vi "PCert-Container-UI.vi"(11 "error constant":errorcluster) -> (15 "error constant 2":errorcluster)   [LabVIEW 2013, in "PCert-Container-UI.lvclass"]
uses:
  PCert-Container-UI.lvclass
  PCert-Container-UI.lvclass/PCert-Container-UI.ctl
  ftw-dataflow/Actor/src/Connector/FTW-ActorConnector.lvclass
  ftw-dataflow/Actor/src/Message/Request/FTW-Message-IncomingRequest.lvclass
  ERP-Glue/PCert-Glue-TreeItem.ctl
  Actors/Globals/Global-SystemSettings.vi
  ftw-dataflow/Actor/src/Instance/FTW-ActorInstance.lvclass
  ftw-dataflow/Actor/src/Ether/FTW-Ether.lvclass
  ERP-ConfigPageNewFeather/PCert-ConfigPageNF.lvclass
  <resource>/Framework/Providers/Wirebird Labs LLC/Deploy/Support/Update Service/Deploy-UpdateService.lvclass
panel:
  in  "UI_Tree_Navigation":string(tree) caption="Navigation Tree"
  in  "Shutdown":bool
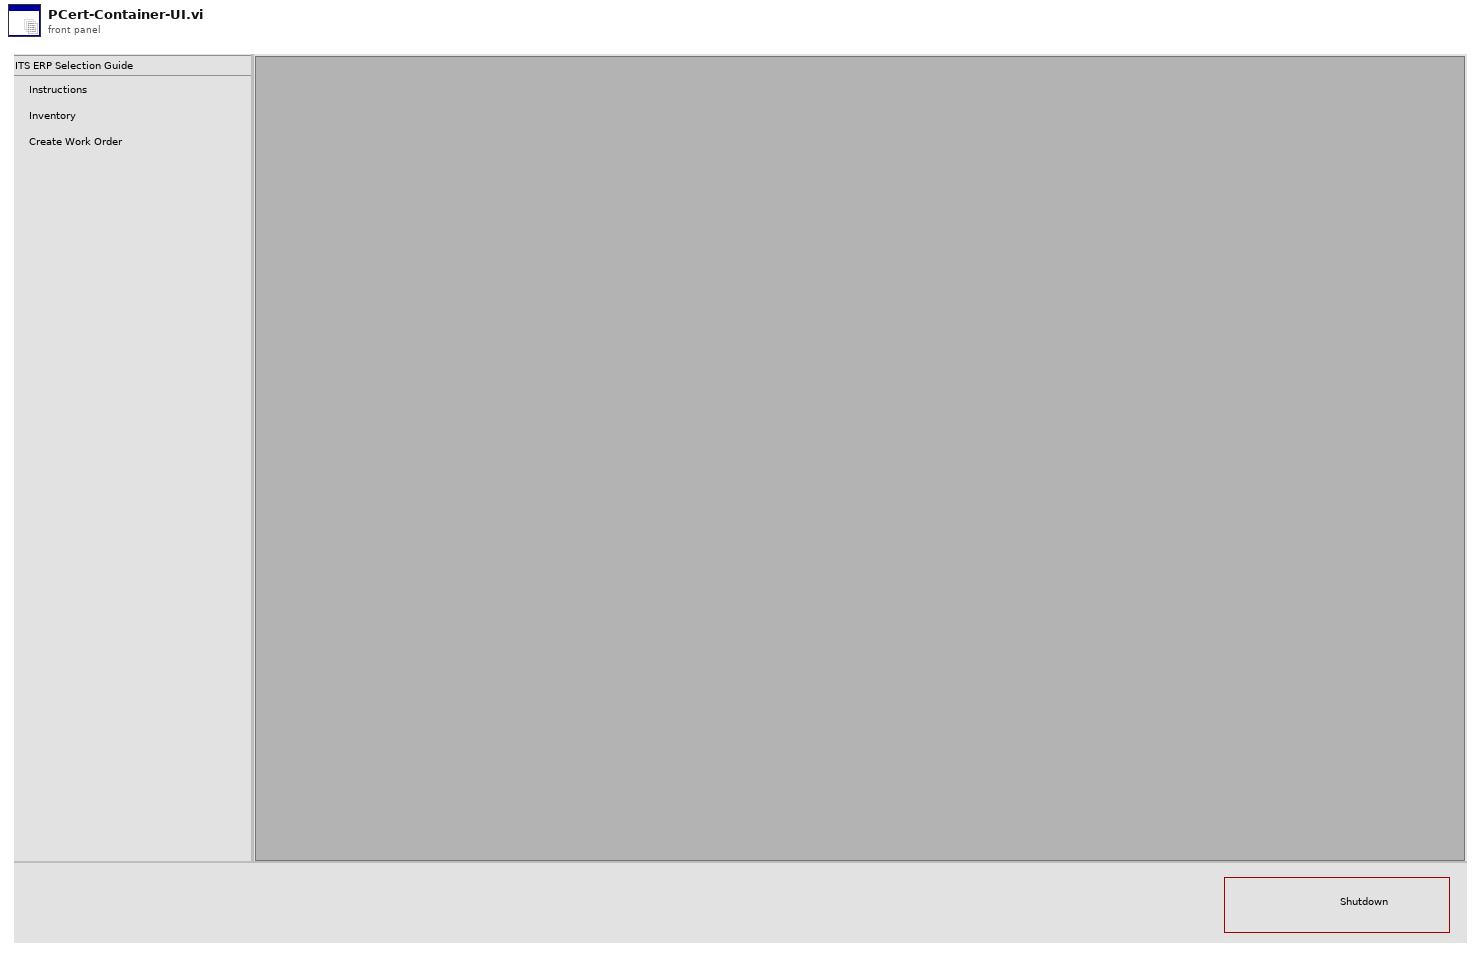
[diagram p1: front panel]
types:
  T1 = typedef "PCert-Glue-TreeItem.ctl" = cluster{"Tag":string, "Parent":string, "Add to Top of Parent":bool, "Type":string, "Indent":i32, "Child Only":bool, "First Cell":string, "Next Cells":string[]}
  T2 = cluster{"Incoming Requests":refnum<event-registration>, "Update Service Event Registration":refnum<event-registration>}
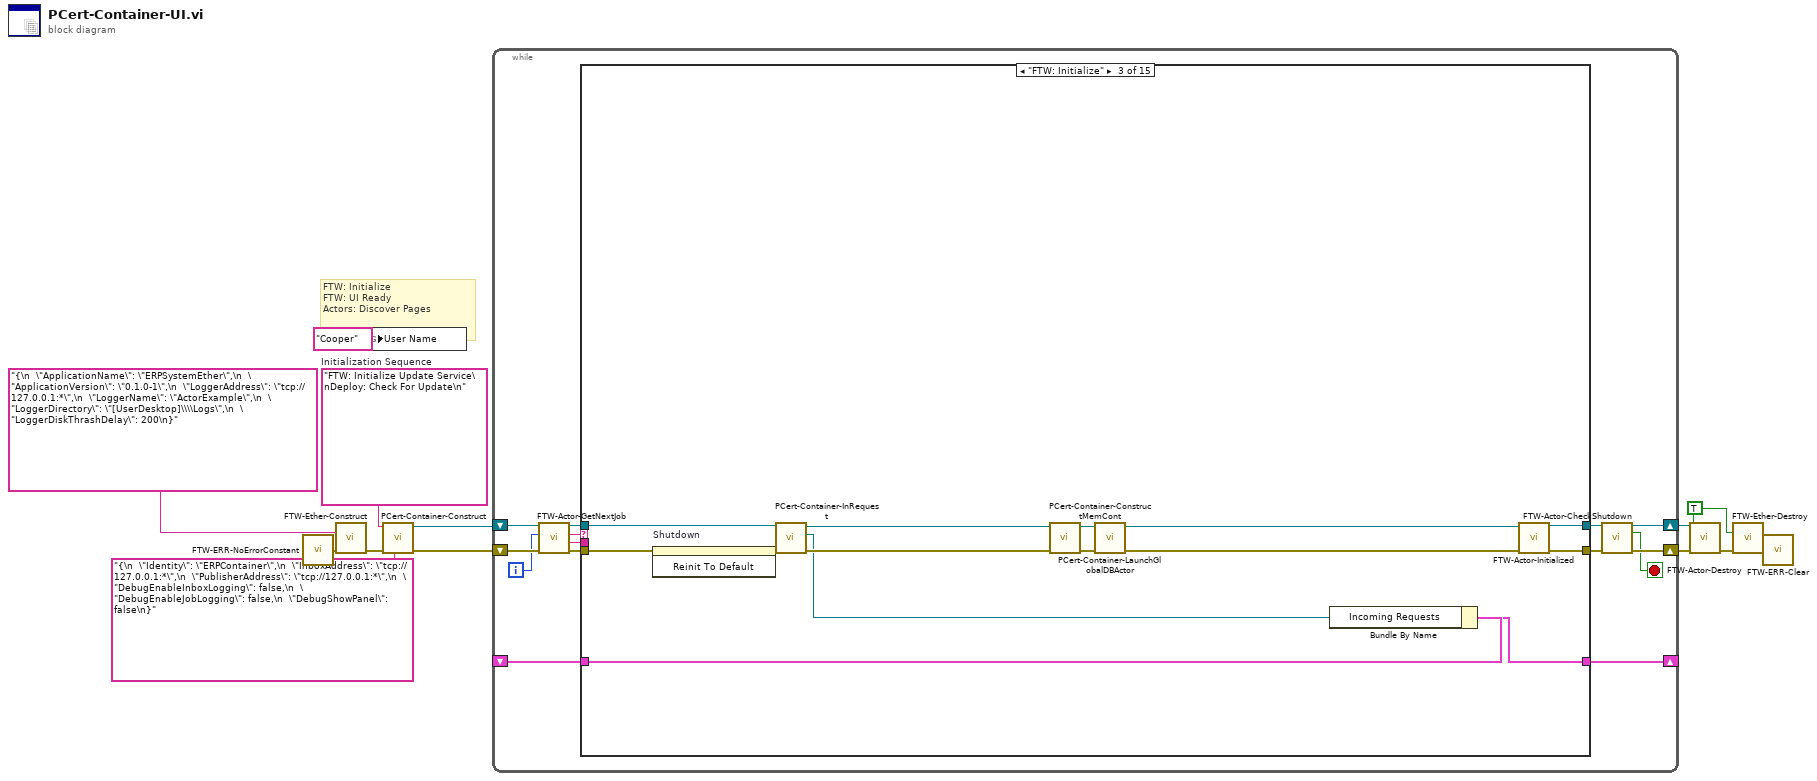
[diagram p0: block diagram]
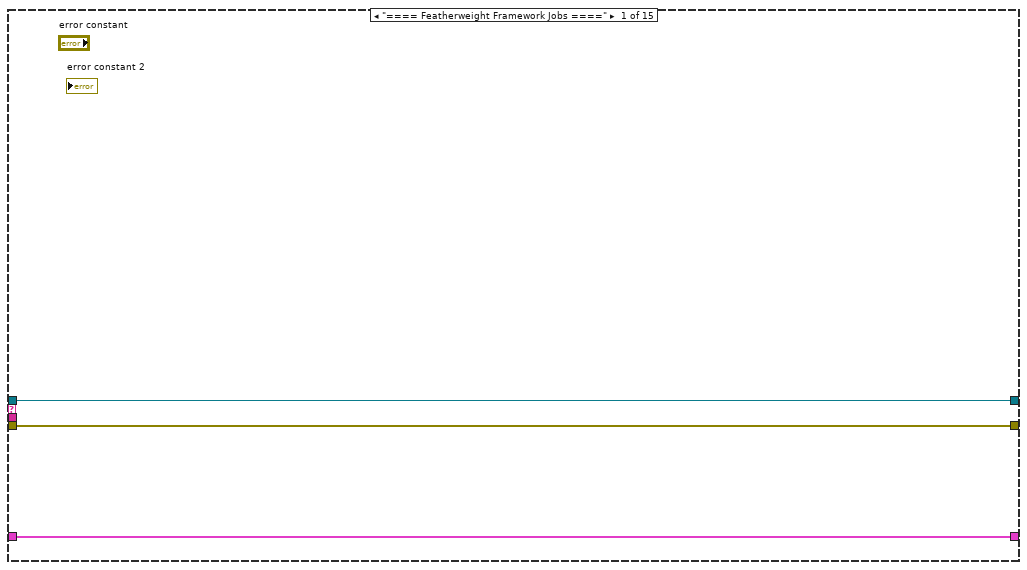
[diagram p2: hidden frame]
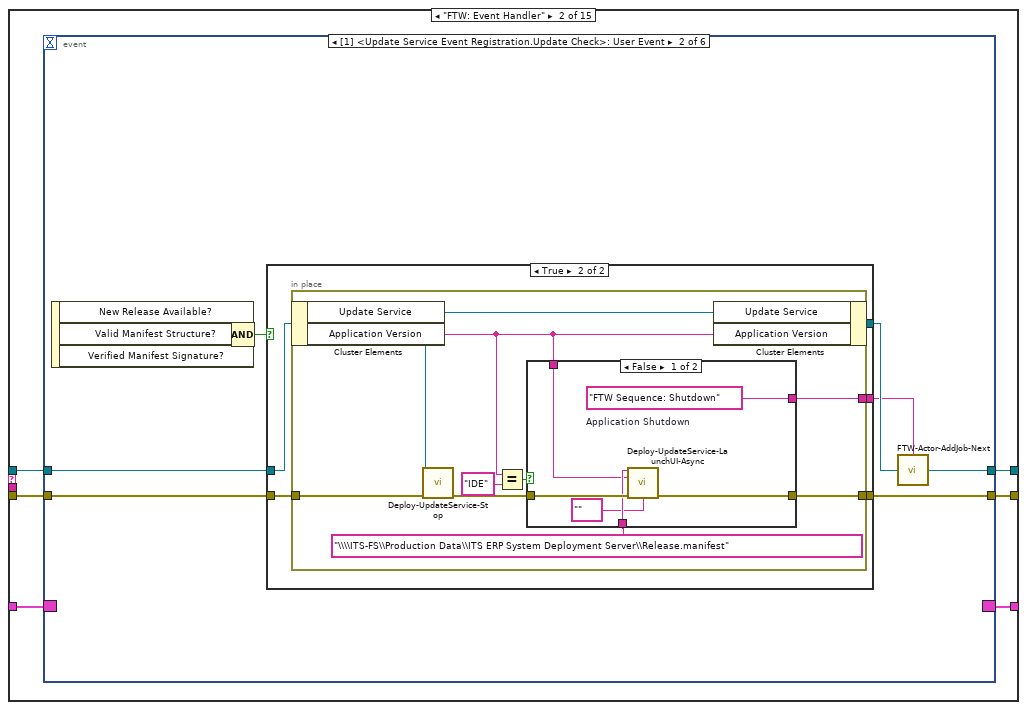
[diagram p3: hidden frame]
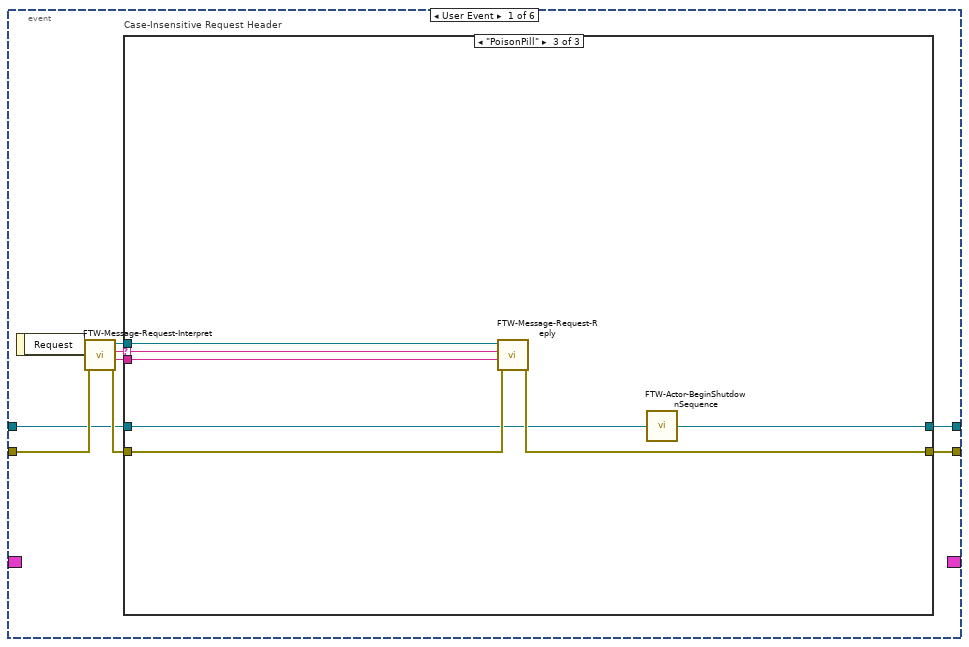
[diagram p4: hidden frame]
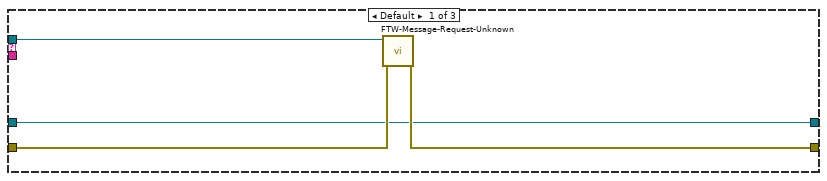
[diagram p5: hidden frame]
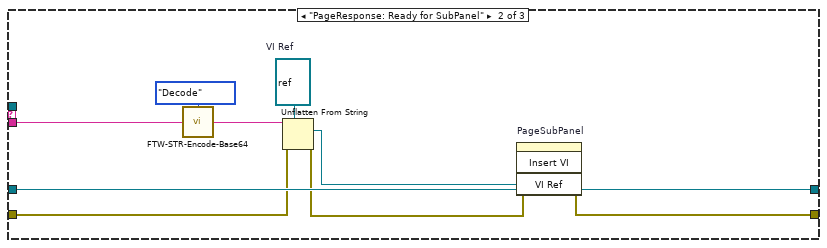
[diagram p6: hidden frame]
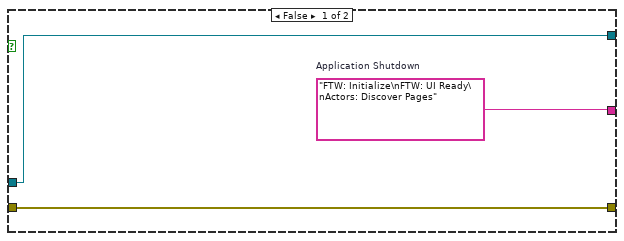
[diagram p7: hidden frame]
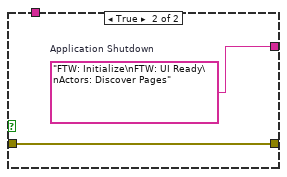
[diagram p8: hidden frame]
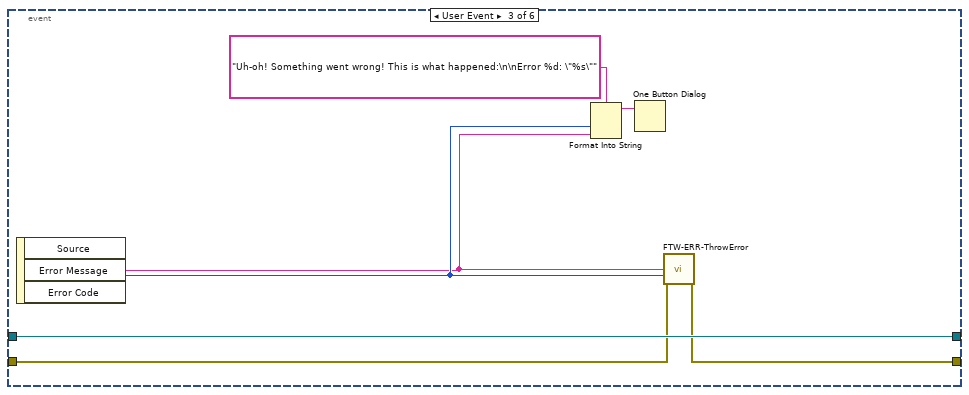
[diagram p9: hidden frame]
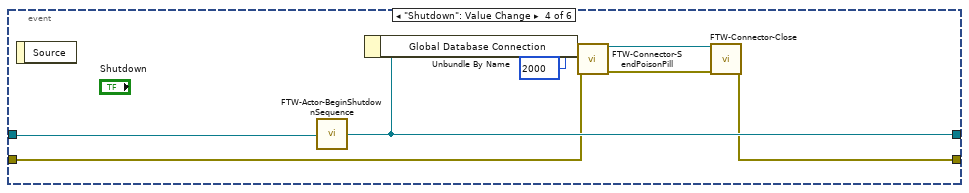
[diagram p10: hidden frame]
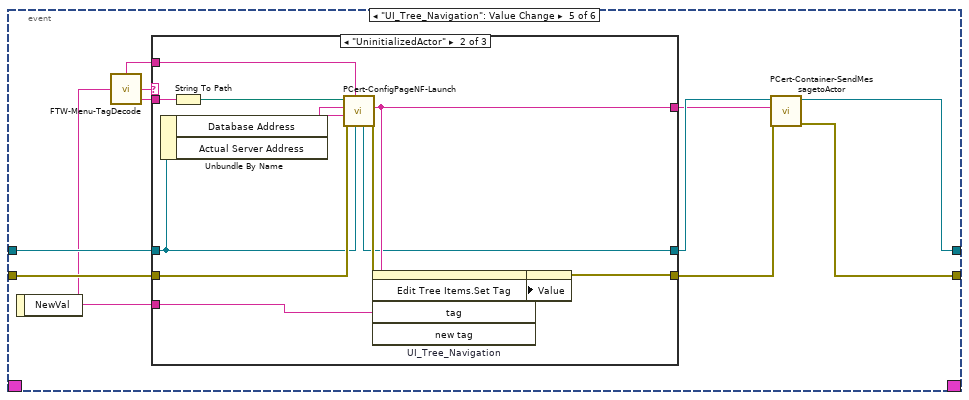
[diagram p11: hidden frame]
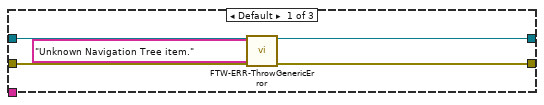
[diagram p12: hidden frame]
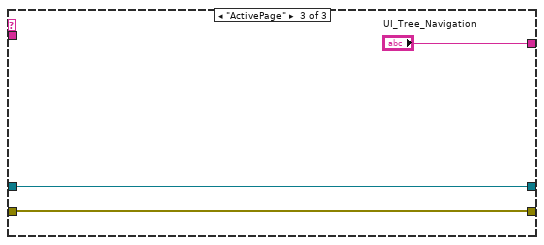
[diagram p13: hidden frame]
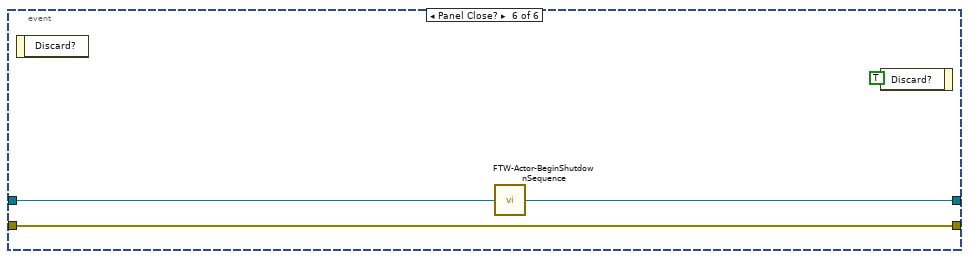
[diagram p14: hidden frame]
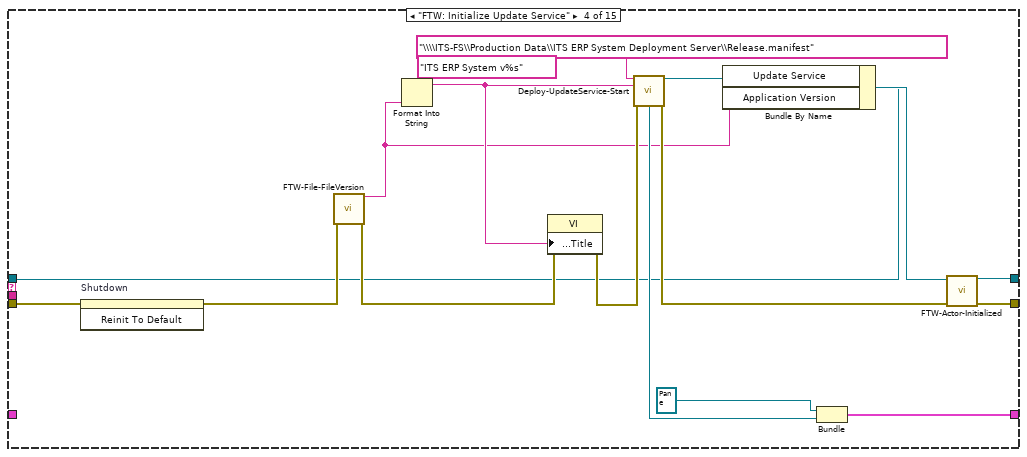
[diagram p15: hidden frame]
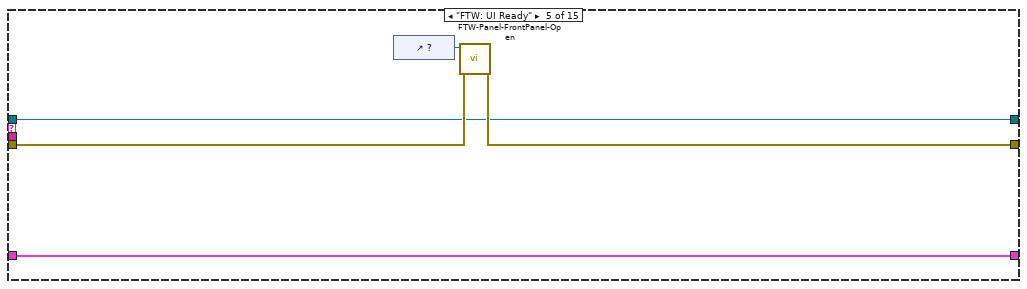
[diagram p16: hidden frame]
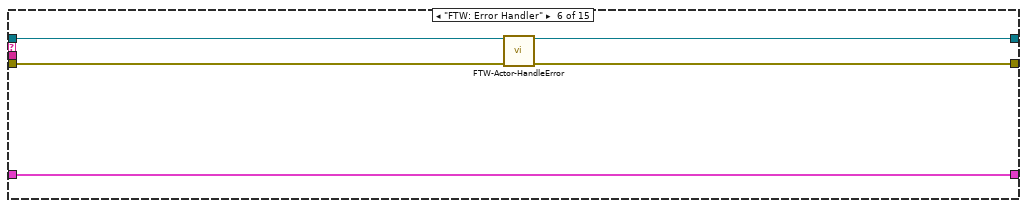
[diagram p17: hidden frame]
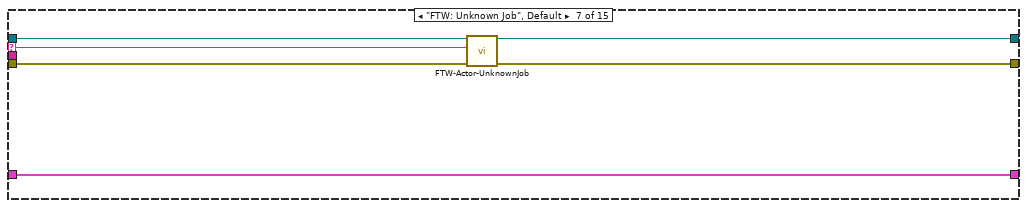
[diagram p18: hidden frame]
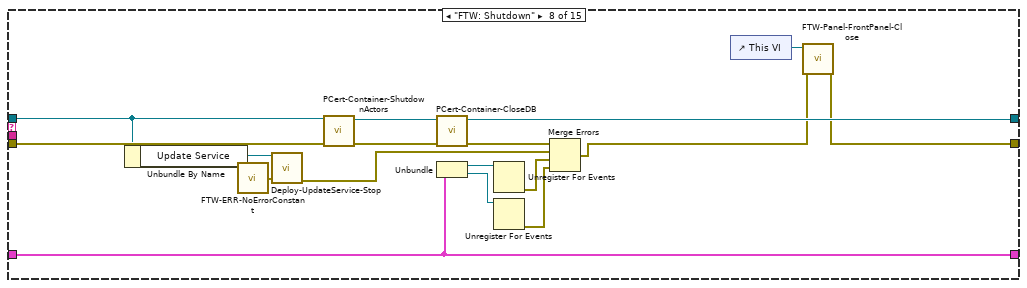
[diagram p19: hidden frame]
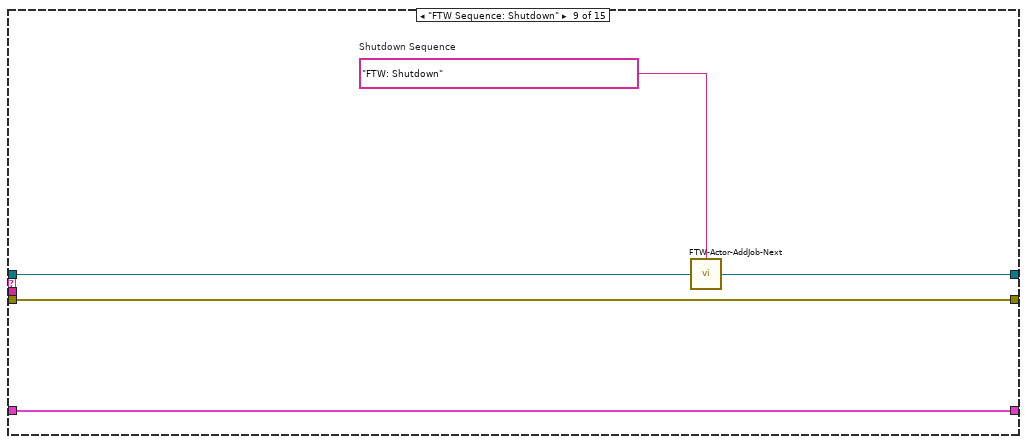
[diagram p20: hidden frame]
diagram:
  w2 = TRUE ("Force Destroy?")
  w6 = "FTW: Initialize Update Service\nDeploy: Check For Update\n"  # Initialization Sequence
  # "FTW: Initialize\nFTW: UI Ready\nActors: Discover Pages"
  n1 = call "FTW-ERR-NoErrorConstant.vi"() -> ("no error"=w4:errorcluster)
  n2 = call "FTW-Ether-Construct.vi"("FTW Ether Configuration"="{\n  \"ApplicationName\": \"ERPSystemEther\",\n  \"ApplicationVersion\": \"0.1.0-1\",\n  \"LoggerAddress\": \"tcp://127.0.0.1:*\",\n  \"LoggerName\": \"ActorExample\",\n  \"LoggerDirectory\": \"[UserDesktop]\\\\Logs\",\n  \"LoggerDiskThrashDelay\": 200\n}", "error in"=w4) -> ("error out"=w5:errorcluster)  [unwired: 13 in]
  n3 = global write "Global-SystemSettings.vi" "User Name"("Cooper" ("User Name")) -> ()
  n4 = call "PCert-Container-Construct.vi"("FTW Actor Instance Configuration"="{\n  \"Identity\": \"ERPContainer\",\n  \"InboxAddress\": \"tcp://127.0.0.1:*\",\n  \"PublisherAddress\": \"tcp://127.0.0.1:*\",\n  \"DebugEnableInboxLogging\": false,\n  \"DebugEnableJobLogging\": false,\n  \"DebugShowPanel\": false\n}", "error in (no error)"=w5, "Initialization Sequence"=w6) -> ("error out"=w8:errorcluster, "ERP-Container-UI out"=w9:refnum<class "PCert-Container-UI.lvclass">)  [unwired: 7 in]
  n5 = while {
    shift-right: [w18] -> w12
    shift-left: w8 -> [w25]
    shift-right: [w15] -> _
    shift-left: _ -> [w14]
    shift-right: [w20] -> w13
    shift-left: w9 -> [w27]
    i -> [w16]
    stop <- w17 stop-if-true
    n6 = call "FTW-Actor-GetNextJob.vi"("error in"=w25, "Jobs Performed"=w16, "FTW Actor Instance"=w27) -> ("error out"=w24:errorcluster, "Job Data"=w22:string, "Job Name"=w23:string, "FTW Actor Instance out"=w26:refnum<class "PCert-Container-UI.lvclass">)  [unwired: 5 in]
    n7 = case shown="\"FTW: Initialize\"" w23 {
      selector: w23 -> [_ _ _ _ _ _ w193 _ _ _ _ _ _ _ _]
      tunnel: [w29 w36 w164 w181 w185 w189 w196 w207 w216 w224 w228 w231 w234 w255 w259] -> w19
      tunnel: w24 -> [w29 w35 w158 w179 w187 w188 w197 w206 w216 w224 w228 w231 w245 w255 w260]
      tunnel: w14 -> [w30 w31 w154 _ w183 w192 w198 w215 w220 w225 w227 w230 w247 w254 w262]
      tunnel: [w30 w32 w152 w180 w183 w192 w198 w215 w220 w225 w227 w230 w247 w254 w262] -> w15
      tunnel: w22 -> [_ _ _ _ _ _ _ _ _ _ _ _ _ _ _]
      tunnel: [w28 w34 w165 w182 w184 w190 w194 w212 w218 w222 w226 w229 w246 w253 w257] -> w21
      tunnel: w26 -> [w28 w33 w161 w169 w184 w191 w195 w202 w219 w223 w226 w229 w246 w253 w261]
      frame "==== Featherweight Framework Jobs ====" {
      }
      frame "FTW: Event Handler" {
        n8 = event shown="[1] <Update Service Event Registration.Update Check>: User Event" {
          selector: w31 -> [_ _ _ _ _ _]
          dyn-events: [_ _ _ _ _ _] -> w32
          timeout: _ -> [_ _ _ _ _ _]
          tunnel: [w42 w69 w103 w113 w118 w150] -> w36
          tunnel: w35 -> [w43 w74 w104 w108 w123 w150]
          tunnel: [w41 w66 w107 w114 w117 w148] -> w34
          tunnel: w33 -> [w40 w75 w107 w115 w124 w149]
          event User Event {
            n9 = event-data() -> ("Request"=w44:refnum<class "FTW-Message-IncomingRequest.lvclass">)  [unwired: 1 in]
            n10 = call "FTW-Message-Request-Interpret.vi"("error in"=w43, "FTW Incoming Request"=w44) -> ("error out"=w45:errorcluster, "Request Body"=w38:string, "Request Header"=w39:string, "FTW Incoming Request out"=w37:refnum<class "FTW-Message-IncomingRequest.lvclass">)  [unwired: 6 in]
            n11 = case "Case-Insensitive Request Header" shown="\"PoisonPill\"" w39 {
              selector: w39 -> [_ _ w61]
              tunnel: [w48 w54 w63] -> w42
              tunnel: w45 -> [w49 w53 w64]
              tunnel: [w46 w58 w65] -> w41
              tunnel: w40 -> [w46 w58 w62]
              tunnel: w38 -> [_ w52 w60]
              tunnel: w37 -> [w47 _ w59]
              frame Default {
                n12 = call "FTW-Message-Request-Unknown.vi"("error in"=w49, "FTW Incoming Request"=w47) -> ("error out"=w48:errorcluster)  [unwired: 9 in]
              }
              frame "PageResponse: Ready for SubPanel" {
                w57 = refnum<vi> refnum  # VI Ref
                n13 = call "FTW-STR-Encode-Base64.vi"("Input"=w52, "Direction"=enum16{"Encode", "Decode"}."Decode") -> ("Output"=w50:string)
                n14 = Unflatten From String(type=w57, binary string=w50, error in (no error)=w53) -> (value=w56:refnum<vi>, error out=w55:errorcluster)  [unwired: 2 in, 1 out]
                n15 = invoke on="PageSubPanel" class="SubPnl" method="Insert VI"(error in=w55, "VI Ref"=w56) -> (error out=w54:errorcluster)  [unwired: 2 in, 3 out]
              }
              frame "PoisonPill" {
                n16 = call "FTW-Message-Request-Reply.vi"("error in"=w64, "Response Body"=w60, "Response Header"=w61, "FTW Incoming Request"=w59) -> ("error out"=w63:errorcluster)  [unwired: 6 in, 1 out]
                n17 = call "FTW-Actor-BeginShutdownSequence.vi"("FTW Actor Instance"=w62) -> ("FTW Actor Instance out"=w65:refnum<class "PCert-Container-UI.lvclass">)  [unwired: 3 in]
              }
            }
          }
          event User Event {
            n18 = event-data() -> ("New Release Available?"=w73:bool, "Valid Manifest Structure?"=w72:bool, "Verified Manifest Signature?"=w71:bool)  [unwired: 1 in]
            n19 = Compound Arithmetic op=AND(w73, w72, w71) -> (w70:bool)
            n20 = case shown="True" w70 {
              tunnel: w75 -> [w78 w83]
              tunnel: w74 -> [w77 w82]
              tunnel: [w78 w81] -> w68
              tunnel: [w77 w80] -> w69
              tunnel: [w76 w79] -> w67
              frame False {
                w76 = "FTW: Initialize\nFTW: UI Ready\nActors: Discover Pages"  # Application Shutdown
              }
              frame True {
                n21 = in-place {
                  in-place-border: w82 -> [w92]
                  in-place-border: [w88] -> w80
                  in-place-border: [w84] -> w79
                  n22 = in-place-cluster #1(w83) -> ("Update Service"=w91:refnum<class "Deploy-UpdateService.lvclass">, "Application Version"=w86:string)
                  n23 = call <resource>:"Deploy-UpdateService-Stop.vi"("Update Service"=w91, "error in"=w92) -> ("error out"=w90:errorcluster)  [unwired: 13 in]
                  n24 = Equal?(x=w86, y="IDE") -> (x = y?=w87:bool)
                  n25 = case shown="False" w87 {
                    tunnel: w90 -> [w98 w100]
                    tunnel: "\\\\ITS-FS\\Production Data\\ITS ERP System Deployment Server\\Release.manifest" ("Manifest URI") -> [w97 _]
                    tunnel: [w95 w100] -> w88
                    tunnel: w86 -> [w94 _]
                    tunnel: [w93 w99] -> w84
                    frame False {
                      w93 = "FTW Sequence: Shutdown"  # Application Shutdown
                      n26 = call <resource>:"Deploy-UpdateService-LaunchUI-Async.vi"("Manifest URI"=w97, "Current Release Version"=w94, "error in"=w98, "Installer Command Line Parameters"="") -> ("error out"=w95:errorcluster)  [unwired: 10 in, 1 out]
                    }
                    frame True {
                      w99 = "FTW: Initialize\nFTW: UI Ready\nActors: Discover Pages"  # Application Shutdown
                    }
                  }
                  n27 = in-place-cluster #1("Update Service"=w91, "Application Version"=w86) -> (w81:refnum<class "PCert-Container-UI.lvclass">)
                }
              }
            }
            n28 = call "FTW-Actor-AddJob-Next.vi"("Add Next in Job Queue"=w67, "FTW Actor Instance"=w68) -> ("FTW Actor Instance out"=w66:refnum<class "PCert-Container-UI.lvclass">)  [unwired: 2 in]
          }
          event User Event {
            n29 = event-data() -> ("Error Message"=w101:string, "Error Code"=w102:i32)  [unwired: 1 in, 1 out]
            n30 = Format Into String(format string="Uh-oh! Something went wrong! This is what happened:\n\nError %d: \"%s\"", w102, w101) -> (resulting string=w106:string)  [unwired: 2 in, 1 out]
            n31 = One Button Dialog(message=w106) -> ()  [unwired: 1 in, 1 out]
            n32 = call "FTW-ERR-ThrowError.vi"("Error Message"=w101, "Error Code"=w102, "error in"=w104) -> ("error out"=w103:errorcluster)  [unwired: 12 in]
          }
          event "Shutdown": Value Change {
            n33 = event-data() -> ()  [unwired: 1 in, 1 out]
            n34 = call "FTW-Actor-BeginShutdownSequence.vi"("FTW Actor Instance"=w115) -> ("FTW Actor Instance out"=w114:refnum<class "PCert-Container-UI.lvclass">)  [unwired: 3 in]
            n35 = Unbundle By Name(w114) -> ("Global Database Connection"=w112:refnum<class "FTW-ActorConnector.lvclass">)
            n36 = call-dynamic "FTW-Connector-SendPoisonPill.vi"("FTW Actor Connector"=w112, "Timeout"=2000, "error in"=w108) -> ("FTW Actor Connector out"=w111:refnum<class "FTW-ActorConnector.lvclass">, "error out"=w110:errorcluster)  [unwired: 8 in, 3 out]
            n37 = call-dynamic "FTW-Connector-Close.vi"("FTW Actor Connector"=w111, "error in"=w110) -> ("error out"=w113:errorcluster)  [unwired: 13 in]
          }
          event "UI_Tree_Navigation": Value Change {
            n38 = event-data() -> ("NewVal"=w122:string)  [unwired: 1 in]
            n39 = call "FTW-Menu-TagDecode.vi"("Menu Item Tag"=w122) -> ("Actor Name"=w116:string, "Command"=w126:string, "Payload"=w125:string)  [unwired: 1 out]
            n40 = case shown="\"UninitializedActor\"" w126 {
              tunnel: w125 -> [_ w142 _]
              tunnel: w124 -> [w130 w135 w146]
              tunnel: [w130 w131 w146] -> w121
              tunnel: w123 -> [w129 w144 w145]
              tunnel: [w128 w132 w145] -> w119
              tunnel: w122 -> [_ w139 _]
              tunnel: [_ w133 "UI_Tree_Navigation"] -> w120
              tunnel: w116 -> [_ w136 _]
              frame Default {
                n41 = call "FTW-ERR-ThrowGenericError.vi"("Error Message"="Unknown Navigation Tree item.", "error in"=w129) -> ("error out"=w128:errorcluster)  [unwired: 13 in]
              }
              frame "UninitializedActor" {
                n42 = Unbundle By Name(w135) -> ("Database Address"=w134:string, "Actual Server Address"=w143:string)
                n43 = String To Path(string=w142) -> (path=w141:path)
                n44 = call "PCert-ConfigPageNF-Launch.vi"("ERP-Container-UI in"=w135, "Actor Name"=w136, "error in (no error)"=w144, "Container Address"=w143, "Database Address"=w134, "Configuration Page VI Filepath"=w141) -> ("error out"=w140:errorcluster, "PageID"=w133:string, "ERP-Container-UI out"=w131:refnum<class "PCert-Container-UI.lvclass">)  [unwired: 3 in]
                n45 = invoke on="UI_Tree_Navigation" class="Tree (strict)" method="Edit Tree Items.Set Tag"(error in=w140, "tag"=w139, "new tag"=w133) -> (error out=w138:errorcluster, "Edit Tree Items:Set Tag"=w137:string)  [unwired: 2 in, 3 out]
                n46 = property on="UI_Tree_Navigation" class="Tree (strict)"(error in=w138, "Value"=w137) -> (error out=w132:errorcluster)  [unwired: 1 in, 1 out]
              }
              frame "ActivePage" {
              }
            }
            n47 = call "PCert-Container-SendMessagetoActor.vi"("error in (no error)"=w119, "ActorID"=w120, "ERP-Container-UI in"=w121) -> ("error out"=w118:errorcluster, "ERP-Container-UI out"=w117:refnum<class "PCert-Container-UI.lvclass">)  [unwired: 7 in]
          }
          event Panel Close? {
            n48 = event-data() -> ()  [unwired: 1 in, 1 out]
            n49 = call "FTW-Actor-BeginShutdownSequence.vi"("FTW Actor Instance"=w149) -> ("FTW Actor Instance out"=w148:refnum<class "PCert-Container-UI.lvclass">)  [unwired: 3 in]
            n50 = event-data("Discard?"=TRUE) -> ()  [unwired: 1 in, 1 out]
          }
        }
      }
      frame "FTW: Initialize" {
        n51 = invoke on="Shutdown" class="Bool (strict)" method="Reinit To Default"(error in=w158) -> (error out=w157:errorcluster)  [unwired: 2 in, 2 out]
        n52 = call "PCert-Container-InRequest.vi"("error in (no error)"=w157, "ERP-Container-UI in"=w161) -> ("error out"=w162:errorcluster, "Incoming Requests"=w153:refnum<event-registration>, "ERP-Container-UI out"=w163:refnum<class "PCert-Container-UI.lvclass">)  [unwired: 7 in]
        n53 = call "PCert-Container-ConstructMemCont.vi"("error in (no error)"=w162, "ERP-Container-UI in"=w163) -> ("error out"=w159:errorcluster, "ERP-Container-UI out"=w160:refnum<class "PCert-Container-UI.lvclass">)  [unwired: 8 in]
        n54 = call "PCert-Container-LaunchGlobalDBActor.vi"("error in (no error)"=w159, "ERP-Container-UI in"=w160) -> ("error out"=w156:errorcluster, "ERP-Container-UI out"=w155:refnum<class "PCert-Container-UI.lvclass">)  [unwired: 8 in]
        n55 = Bundle By Name(cluster=w154, "Incoming Requests"=w153) -> (w152:T2)
        n56 = call-dynamic "FTW-Actor-Initialized.vi"("FTW Actor Instance"=w155, "error in"=w156) -> ("FTW Actor Instance out"=w165:refnum<class "PCert-Container-UI.lvclass">, "error out"=w164:errorcluster)  [unwired: 12 in]
      }
      frame "FTW: Initialize Update Service" {
        n57 = invoke on="Shutdown" class="Bool (strict)" method="Reinit To Default"(error in=w179) -> (error out=w170:errorcluster)  [unwired: 2 in, 2 out]
        n58 = call "FTW-File-FileVersion.vi"("error in"=w170) -> ("File Version"=w166:string, "error out"=w176:errorcluster)  [unwired: 10 in, 3 out]
        n59 = Format Into String(format string="ITS ERP System v%s", w166) -> (resulting string=w167:string)  [unwired: 2 in, 1 out]
        n60 = property class="VI"(error in=w176, "Front Panel.Title"=w167) -> (error out=w175:errorcluster)  [unwired: 1 in, 1 out]
        n61 = call <resource>:"Deploy-UpdateService-Start.vi"("Manifest URI"="\\\\ITS-FS\\Production Data\\ITS ERP System Deployment Server\\Release.manifest", "Current Release Version"=w167, "error in"=w175) -> ("Update Service"=w172:refnum<class "Deploy-UpdateService.lvclass">, "Update Service Event Registration"=w174:refnum<event-registration>, "error out"=w173:errorcluster)  [unwired: 10 in]
        n62 = Bundle By Name(cluster=w169, "Update Service"=w172, "Application Version"=w166) -> (w171:refnum<class "PCert-Container-UI.lvclass">)
        n63 = Bundle("Incoming Requests"=refnum<event-registration> refnum, "Update Service Event Registration"=w174) -> (w180:T2)  [unwired: 1 in]
        n64 = call-dynamic "FTW-Actor-Initialized.vi"("FTW Actor Instance"=w171, "error in"=w173) -> ("FTW Actor Instance out"=w182:refnum<class "PCert-Container-UI.lvclass">, "error out"=w181:errorcluster)  [unwired: 12 in]
      }
      frame "FTW: UI Ready" {
        n65 = control-ref of="?"() -> (w186:refnum<vi>)
        n66 = call "FTW-Panel-FrontPanel-Open.vi"("error in"=w187, "VI Ref"=w186) -> ("error out"=w185:errorcluster)  [unwired: 8 in, 1 out]
      }
      frame "FTW: Error Handler" {
        n67 = call-dynamic "FTW-Actor-HandleError.vi"("FTW Actor Instance"=w191, "error in"=w188) -> ("FTW Actor Instance out"=w190:refnum<class "PCert-Container-UI.lvclass">, "error out"=w189:errorcluster)  [unwired: 11 in, 1 out]
      }
      frame "FTW: Unknown Job", Default {
        n68 = call-dynamic "FTW-Actor-UnknownJob.vi"("FTW Actor Instance"=w195, "Unknown Job"=w193, "error in"=w197) -> ("FTW Actor Instance out"=w194:refnum<class "PCert-Container-UI.lvclass">, "error out"=w196:errorcluster)  [unwired: 11 in]
      }
      frame "FTW: Shutdown" {
        n69 = Unbundle By Name(w202) -> ("Update Service"=w201:refnum<class "Deploy-UpdateService.lvclass">)
        n70 = call "FTW-ERR-NoErrorConstant.vi"() -> ("no error"=w200:errorcluster)
        n71 = call <resource>:"Deploy-UpdateService-Stop.vi"("Update Service"=w201, "error in"=w200) -> ("error out"=w199:errorcluster)  [unwired: 13 in]
        n72 = call "PCert-Container-ShutdownActors.vi"("error in (no error)"=w206, "ERP-Container-UI in"=w202) -> ("error out"=w210:errorcluster, "ERP-Container-UI out"=w211:refnum<class "PCert-Container-UI.lvclass">)  [unwired: 8 in]
        n73 = call "PCert-Container-CloseDB.vi"("error in (no error)"=w210, "ERP-Container-UI in"=w211) -> ("error out"=w209:errorcluster, "ERP-Container-UI out"=w212:refnum<class "PCert-Container-UI.lvclass">)  [unwired: 8 in]
        n74 = Unbundle(w215) -> ("Incoming Requests"=w214:refnum<event-registration>, "Update Service Event Registration"=w204:refnum<event-registration>)
        n75 = Unregister For Events(event registration refnum=w214) -> (error out=w213:errorcluster)  [unwired: 1 in]
        n76 = Unregister For Events(event registration refnum=w204) -> (error out=w203:errorcluster)  [unwired: 1 in]
        n77 = Merge Errors(w209, w199, w213, w203) -> (w208:errorcluster)
        n78 = control-ref of="This VI"() -> (w205:refnum<vi>)
        n79 = call "FTW-Panel-FrontPanel-Close.vi"("error in"=w208, "VI Ref"=w205) -> ("error out"=w207:errorcluster)  [unwired: 8 in, 1 out]
      }
      frame "FTW Sequence: Shutdown" {
        w217 = "FTW: Shutdown"  # Shutdown Sequence
        n80 = call "FTW-Actor-AddJob-Next.vi"("Add Next in Job Queue"=w217, "FTW Actor Instance"=w219) -> ("FTW Actor Instance out"=w218:refnum<class "PCert-Container-UI.lvclass">)  [unwired: 2 in]
      }
      frame "==== Actor-Specific Job Sequences ====" {
        w221 = ""  # Job Sequence
        n81 = call "FTW-Actor-AddJob-Next.vi"("Add Next in Job Queue"=w221, "FTW Actor Instance"=w223) -> ("FTW Actor Instance out"=w222:refnum<class "PCert-Container-UI.lvclass">)  [unwired: 2 in]
      }
      frame "==== Application Logic ====" {
      }
      frame "Actors: Launch Global DB Actor" {
      }
      frame "Actors: Discover Pages" {
        # "Make it go to the default page; in the future,\nthis can be replaced by a \"Last Page Visited\""
        n82 = call "PCert-DiscoverActors.vi"("Custom Config Pages Directory"=path "", "error in"=w245) -> ("Display Names"=w244:string[], "Tree Tags"=w237:string[], "error out"=w240:errorcluster)  [unwired: 9 in, 2 out]
        n83 = for {
          tunnel: T1 {"Tag"="", "Parent"="", "Add to Top of Parent"=FALSE, "Type"="", "Indent"=0, "Child Only"=FALSE, "First Cell"="", "Next Cells"=[]} ("Tree Item") -> [w252]
          tunnel: [w251] -> w241 mode=indexing
          tunnel: w237 -> [w248] mode=indexing
          tunnel: w244 -> [w250] mode=indexing
          n84 = Bundle By Name(cluster=w252, "Child Only"=TRUE, "First Cell"=w250, "Tag"=w248) -> (w251:T1)
        }
        n85 = control-ref of="UI_Tree_Navigation"() -> (w242:refnum<vi>)
        n86 = call "PCert-Glue-Tree-AddItems.vi"("Tree Ctl Ref"=w242, "Tree Items to Create"=w241, "Delete Tree Items First?"=TRUE, "Collapse all new items?"=FALSE, "error in"=w240) -> ("error out"=w236:errorcluster)  [unwired: 8 in, 2 out]
        n87 = Index Array(array=w237, index=0) -> (element=w235:string)
        n88 = property on="UI_Tree_Navigation" class="Tree (strict)"(error in=w236, "Val(Sgnl)"=w235) -> (error out=w234:errorcluster)  [unwired: 1 in, 1 out]
      }
      frame "=======Deploy Update Service========" {
      }
      frame "Deploy: Check For Update" {
        n89 = in-place {
          in-place-border: w260 -> [w268]
          in-place-border: [w264] -> w259
          in-place-border: [w263] -> w256
          n90 = in-place-cluster #2(w261) -> ("Update Service"=w270:refnum<class "Deploy-UpdateService.lvclass">, "Application Version"=w265:string)
          n91 = Equal?(x=w265, y="IDE") -> (x = y?=w266:bool)
          n92 = case shown="False" w266 {
            tunnel: [w275 w278] -> w269
            tunnel: [w274 w279] -> w264
            tunnel: w270 -> [w273 w278]
            tunnel: w268 -> [w272 w279]
            tunnel: ["" ("Application Shutdown") w277] -> w263
            frame False {
              n93 = call <resource>:"Deploy-UpdateService-CheckNow.vi"("Update Service"=w273, "Show UI?"=FALSE, "error in"=w272) -> ("Update Service out"=w275:refnum<class "Deploy-UpdateService.lvclass">, "error out"=w274:errorcluster)  [unwired: 11 in]
            }
            frame True {
              w277 = "FTW: Initialize\nFTW: UI Ready\nActors: Discover Pages"  # Application Shutdown
            }
          }
          n94 = in-place-cluster #2("Update Service"=w269, "Application Version"=w265) -> (w258:refnum<class "PCert-Container-UI.lvclass">)
        }
        n95 = call "FTW-Actor-AddJob-Next.vi"("Add Next in Job Queue"=w256, "FTW Actor Instance"=w258) -> ("FTW Actor Instance out"=w257:refnum<class "PCert-Container-UI.lvclass">)  [unwired: 2 in]
      }
    }
    n96 = call "FTW-Actor-CheckShutdown.vi"("FTW Actor Instance"=w21, "error in"=w19) -> ("FTW Actor Instance out"=w20:refnum<class "PCert-Container-UI.lvclass">, "Shutdown?"=w17:bool, "error out"=w18:errorcluster)  [unwired: 11 in]
  }
  n97 = call-dynamic "FTW-Actor-Destroy.vi"("FTW Actor Instance"=w13, "Force Destroy?"=w2, "error in"=w12) -> ("error out"=w11:errorcluster)  [unwired: 12 in]
  n98 = call "FTW-Ether-Destroy.vi"("Force Destroy?"=w2, "error in"=w11) -> ("error out"=w3:errorcluster)  [unwired: 13 in]
  n99 = call "FTW-ERR-Clear.vi"("error to snuff"=w3) -> ()  [unwired: 1 out]
